vi "GlobalCenter.vi"() -> ()   [LabVIEW 2010]
panel:
  out "Center":bool
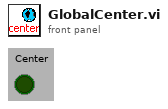
[diagram p1: front panel]
diagram:
